vi "Initialise.vi"(8 "error in (no error)":errorcluster, 10 "Message in":refnum<class "InitialiseMessage.lvclass">, 11 "Trace in":refnum<class "Trace.lvclass">) -> (0 "error out":errorcluster, 3 "Trace out":refnum<class "Trace.lvclass">)   [LabVIEW 2012, in "Trace.lvclass"]
doc: "This method is called when an initialise message is received. It mainly initialises the RabbitMQ connectivity. \n\nOverride this method when your component needs special initialisation (e.g. of software or hardware resources). In that case, don't forget to call the parent for proper implementation. If your component owns subcomponents, they count as resources, so you have to initialise them by calling their own initialise functions"
uses:
  Trace.lvclass
  <vilib>/Distrio/Murmex/InitialiseMessage/InitialiseMessage.lvclass
  <vilib>/Distrio/Murmex/Murmex/Murmex.lvclass
  Trace.lvclass/Trace.ctl
panel:
  # "This method is called when the INTIALISE\ntrigger is sent. \n\nOverride this method when your component needs to\nrespond to this trigger. \n\nCall parent for proper implementation"
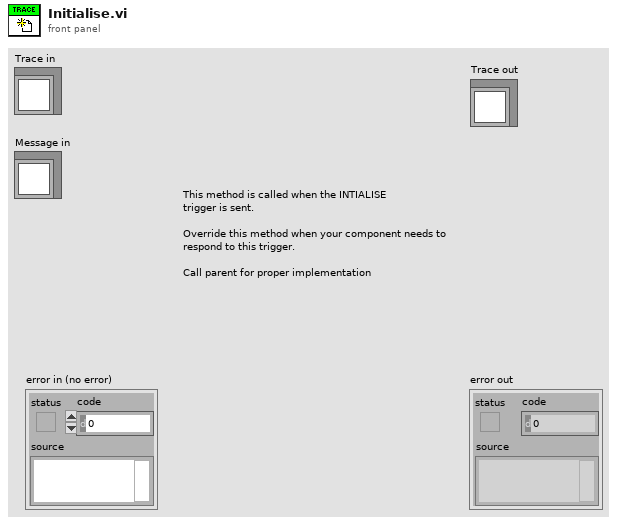
[diagram p1: front panel]
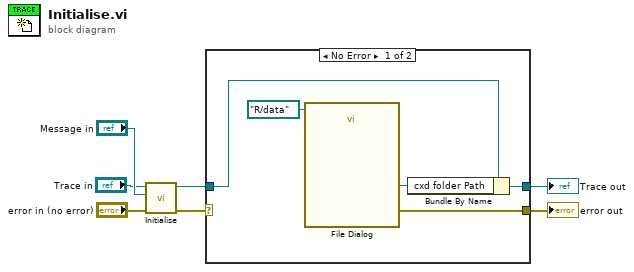
[diagram p0: block diagram]
diagram:
  n1 = call-parent "Initialise.vi"("error in (no error)"="error in (no error)", "Message in"="Message in", "Murmex in"="Trace in") -> ("error out"=w4:errorcluster, "Murmex out"=w3:refnum<class "Trace.lvclass">)  [unwired: 7 in]
  n2 = case shown="No Error" w4 {
    selector: w4 -> [_ w14]
    tunnel: w3 -> [w10 w13]
    tunnel: [w12 w14] -> w2
    tunnel: [w11 w13] -> w1
    frame No Error {
      n3 = call "File Dialog"("start path"=path "R:/data") -> ("selected path"=w9:path, "error out"=w12:errorcluster)  [unwired: 11 in, 2 out]
      n4 = Bundle By Name(cluster=w10, "cxd folder Path"=w9) -> (w11:refnum<class "Trace.lvclass">)
    }
    frame Error {
    }
  }
  "error out" <- w2
  "Trace out" <- w1
